vi "Map out UUID-value lists.vi"(5 "UUIDs to extract":string[](array[string]), 8 "error in":errorcluster, 10 "values in":dbl[](array[numeric]), 11 "UUIDs in":string[](array[string])) -> (0 "error out":errorcluster, 1 "remapped?":bool, 2 "values out":dbl[](array[numeric])=[0.0, 999.0, 2.0, 3.0, nan, 5.0, 6.0, 7.0], 3 "UUIDs out":string[](array[string])=["A", "B", "C", "D", "E", "F", "G"], 6 "values extracted":dbl[](array[numeric])=[999.0, nan])   [LabVIEW 2020]
uses:
  Index Array Elements/Index Array Elements - double.vi
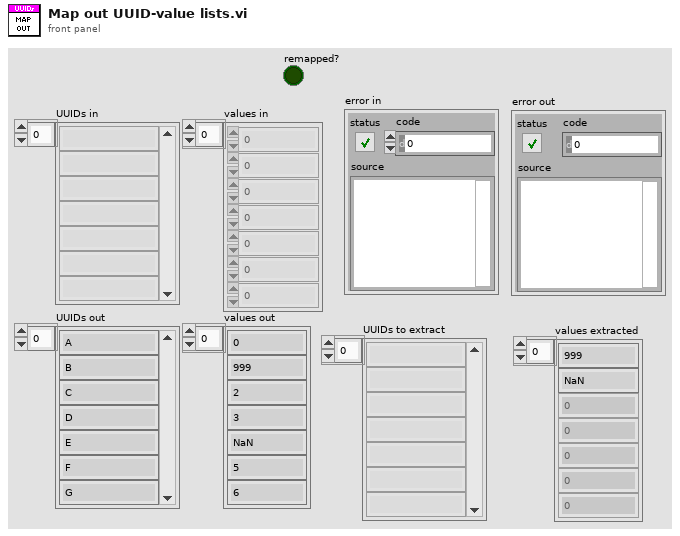
[diagram p1: front panel]
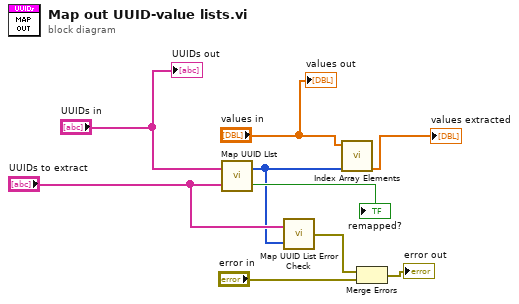
[diagram p0: block diagram]
diagram:
  n1 = call "Map UUID LIst.vi"("UUIDs"="UUIDs to extract", "UUID List"="UUIDs in") -> ("remapped?"=→"remapped?":bool, "indices"=w4:i32[])
  n2 = call "Map UUID List Error Check.vi"("indices"=w4, "UUIDs"="UUIDs to extract") -> ("error constant"=w3:errorcluster)
  n3 = call-poly "Index Array Elements.vi"("indices (none)"=w4, "1D Array"="values in") -> ("output array"=→"values extracted":dbl[])  [unwired: 5 in]
  n4 = Merge Errors(w3, "error in") -> (→"error out":errorcluster)
  "values out" <- "values in"
  "UUIDs out" <- "UUIDs in"
